vi "Choose UI LED Matrix Colors.vi"(7 "Boolean in":refnum<vi>, 8 "error in (no error)":errorcluster, 9 "Color Background":T1(ring), 11 "Color":T1(ring)) -> (0 "error out":errorcluster)   [LabVIEW 2015]
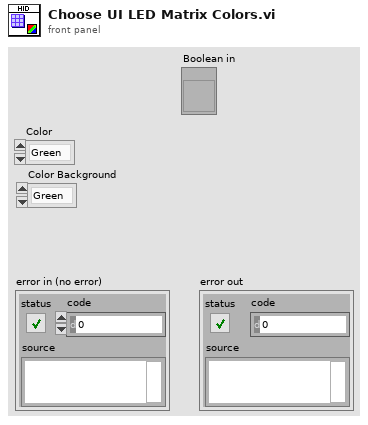
[diagram p1: front panel]
types:
  T1 = enum16{"Green", "Blue", "Red", "White", "Pink", "Yellow", "Turquoise", "Black"}
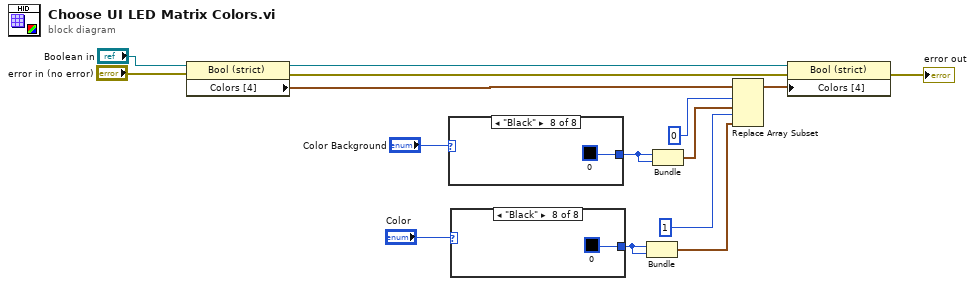
[diagram p0: block diagram]
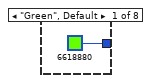
[diagram p2: hidden frame]
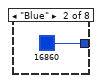
[diagram p3: hidden frame]
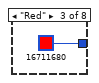
[diagram p4: hidden frame]
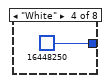
[diagram p5: hidden frame]
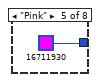
[diagram p6: hidden frame]
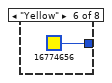
[diagram p7: hidden frame]
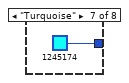
[diagram p8: hidden frame]
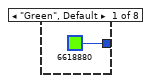
[diagram p9: hidden frame]
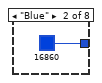
[diagram p10: hidden frame]
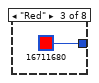
[diagram p11: hidden frame]
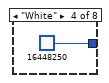
[diagram p12: hidden frame]
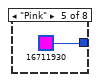
[diagram p13: hidden frame]
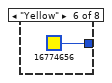
[diagram p14: hidden frame]
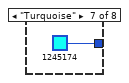
[diagram p15: hidden frame]
diagram:
  n1 = property on="Property Node" class="Bool (strict)"(reference="Boolean in", error in="error in (no error)") -> (reference out=w5:refnum<vi>, error out=w13:errorcluster, "Colors [4]"=w4:cluster{u32, u32}[])
  n2 = case shown="\"Black\"" "Color Background" {
    tunnel: [u32 6618880 ("LED ON Color") u32 16860 ("LED OFF Color") u32 16711680 ("LED ON Color") u32 16448250 ("LED ON Color") u32 16711930 ("LED ON Color") u32 16774656 ("LED ON Color") u32 1245174 ("LED ON Color") u32 0 ("LED ON Color")] -> w11
    frame "Green", Default {
    }
    frame "Blue" {
    }
    frame "Red" {
    }
    frame "White" {
    }
    frame "Pink" {
    }
    frame "Yellow" {
    }
    frame "Turquoise" {
    }
    frame "Black" {
    }
  }
  n3 = case shown="\"Black\"" "Color" {
    tunnel: [u32 6618880 ("LED ON Color") u32 16860 ("LED OFF Color") u32 16711680 ("LED ON Color") u32 16448250 ("LED ON Color") u32 16711930 ("LED ON Color") u32 16774656 ("LED ON Color") u32 1245174 ("LED ON Color") u32 0 ("LED ON Color")] -> w3
    frame "Green", Default {
    }
    frame "Blue" {
    }
    frame "Red" {
    }
    frame "White" {
    }
    frame "Pink" {
    }
    frame "Yellow" {
    }
    frame "Turquoise" {
    }
    frame "Black" {
    }
  }
  n4 = Bundle("LED ON Color"=w3, "LED ON Color"=w3) -> (w2:cluster{"LED ON Color":u32, "LED ON Color":u32})  [unwired: 1 in]
  n5 = Bundle("LED ON Color"=w11, "LED ON Color"=w11) -> (w10:cluster{"LED ON Color":u32, "LED ON Color":u32})  [unwired: 1 in]
  n6 = Replace Array Subset(array=w4, new element #1=w10, index #1=0 ("index"), new element #2=w2, index #2=1 ("index")) -> (w12:cluster{u32, u32}[])
  n7 = property on="Property Node" class="Bool (strict)"(reference=w5, error in=w13, "Colors [4]"=w12) -> (error out=→"error out":errorcluster)  [unwired: 1 out]
